vi "Untitled 12.vi"   [LabVIEW 2019, in "Instrument.lvclass"]
uses:
  Instrument.lvclass
  ce86ec23-ce1a-4ddf-8831-03109916d10e.vi
  245a6bf0-7a94-413a-90f0-5e377c65d7be.vi
  f8c5686a-5e9b-4782-9975-992b5e36aacc.vi
  <vilib>/JDP Science/JSONtext/Make JSON Array.vi
  JSON-RPC/JSON-RPC/private/Write ids.vi
  JSON-RPC/JSON-RPC/private/Read ids.vi
  JSON-RPC/JSON-RPC/private/Parse Response-JSONtext.vi
  f8c5686a-5e9b-4782-9975-992b5e36aacc.vi/b79c4c06-e5f1-4758-ab2c-3fa5ec79f073.vi
  f8c5686a-5e9b-4782-9975-992b5e36aacc.vi/739c1e3f-3a8f-4469-9eb8-add2a6430968.vi
  JSON-RPC/JSON-RPC/private/Parse Response-JSONtext.vi/7ce7fba8-9f44-478d-b6cb-b571ff29f2f5.vi
  JSON-RPC/JSON-RPC/private/Parse Response-JSONtext.vi/8c905beb-ab4c-49e3-b5c6-2c663b7b30d7.vi
  JSON-RPC/JSON-RPC/private/Parse Response-JSONtext.vi/fce5892e-0c40-47e1-88e0-6c122aadefe2.vi
  <vilib>/JDP Science/JSONtext/Find Item.vi
  <vilib>/JDP Science/JSONtext/String Subset.vi
  JSON-RPC/JSON-RPC/private/Create Request-JSONtext.vi
  <vilib>/JDP Science/JSONtext/support/Format JSON Array Text.vi
  JSON-RPC/JSON-RPC/private/Create Response-JSONtext.vi
  <vilib>/JDP Science/JSONtext/JSON type.vi
  <vilib>/JDP Science/JSONtext/Get Array Elements.vi
  <vilib>/JDP Science/JSONtext/Get all Object Items.vi
  <vilib>/JDP Science/JSONtext/Parsing/Parse Full Path or Item Name.vi
  <vilib>/JDP Science/JSONtext/Next JSON Value.vi
  <vilib>/JDP Science/JSONtext/support/Error Cluster From Code.vi
  <vilib>/JDP Science/JSONtext/Offset/Find Item Locations by Path.vi
  <vilib>/JDP Science/JSONtext/JSON text to Variant.vi
  <vilib>/Utility/error.llb/Error Cluster From Error Code.vi
  <vilib>/Utility/Data Type/Get Type Information.vi
  JSON-RPC/JSON-RPC/JSON-RPC.lvclass
  <vilib>/JDP Science/JSONtext/LVClass Serializer/JSONtext LVClass Serializer.lvclass
  <vilib>/addons/_JKI Toolkits/Caraya/classes/Assert/Assert.lvclass
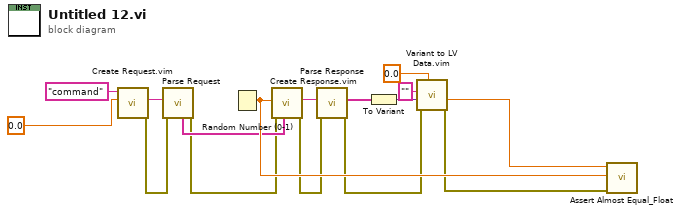
[diagram p0: block diagram]
diagram:
  n1 = call "Create Request.vim"("params"=0.0, "method"="command") -> ("error out"=w2:errorcluster, "{JSON} Requests"=w15:string)  [unwired: 6 in, 2 out]
  n2 = call "Parse Request.vi"("error in (no error)"=w2, "{JSON} Request"=w15) -> ("error out"=w3:errorcluster, "IDs"=w6:string[])  [unwired: 5 in, 3 out]
  n3 = Random Number (0-1)() -> (number: 0 to 1=w8:dbl)
  n4 = call "Create Response.vim"("ids"=w6, "error in (no error)"=w3, "results"=w8) -> ("error out"=w4:errorcluster, "{JSON} Response"=w13:string)  [unwired: 6 in, 1 out]
  n5 = call "Parse Response.vi"("error in (no error)"=w4, "{JSON} Response"=w13) -> ("error out"=w5:errorcluster, "results"=w12:string[])  [unwired: 5 in, 3 out]
  n6 = To Variant(anything=w12) -> (Variant=w11:variant)
  n7 = call "Variant to LV Data.vim"("type"=0.0, "error in (no error)"=w5, "JSON Data in"=w11, "Command"="") -> ("error out"=w1:errorcluster, "Data out"=w10:dbl)  [unwired: 4 in, 2 out]
  n8 = call <vilib>:"Assert Almost Equal_Float.vi"("error in (no error)"=w1, "Y"=w8, "X"=w10) -> ()  [unwired: 8 in, 1 out]
